vi "CreateWindow.vi"(8 "error in (no error)":errorcluster, 10 "Window Type":refnum<class "Window.lvclass">, 11 "Engine in":refnum<class "Engine.lvclass">) -> (0 "error out":errorcluster, 2 "Window Instance":refnum<class "Window.lvclass">, 3 "Engine out":refnum<class "Engine.lvclass">)   [LabVIEW 2020, in "GLF.lvlib" / "Engine.lvclass"]
uses:
  Engine.lvclass
  Engine.lvclass/Engine.ctl
  Window/Window.lvclass
  C:/Users/saukko/Dev/GLF/Sources/GLF/IUseDVRHandler/IUseDVRHandler.lvclass
  C:/Users/saukko/Dev/GLF/Sources/GLF/IAmGLF/IAmGLF.lvclass
  C:/Users/saukko/Dev/GLF/Sources/GLF/Window/Window.lvclass
  IAmGLF/IAmGLF.lvclass
  Command--enum.ctl
  Command-CreateWindow--cluster.ctl
  IAmGLF/InstanciationNotifierData--cluster.ctl
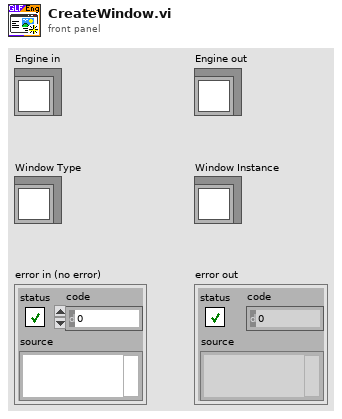
[diagram p1: front panel]
types:
  T1 = typedef "GLF.lvlib/IAmGLF.lvclass/InstanciationNotifierData--cluster.ctl" = cluster{"GLF Instance":refnum<class "IAmGLF.lvclass">, "Error":errorcluster}
  T2 = typedef "GLF.lvlib/Engine.lvclass/Command-CreateWindow--cluster.ctl" = cluster{"Window Type":refnum<class "Window.lvclass">, "Error Return Notifier":refnum<notifier>}
  T3 = typedef "GLF.lvlib/Engine.lvclass/Command--enum.ctl" = enum16{"Quit", "Create Window"}
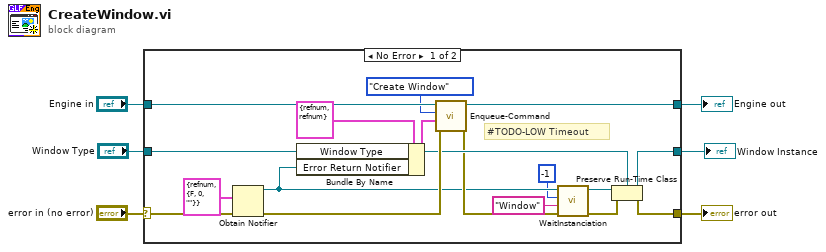
[diagram p0: block diagram]
diagram:
  n1 = case shown="No Error" "error in (no error)" {
    selector: "error in (no error)" -> [w19 w26]
    tunnel: [w9 w26] -> w5
    tunnel: [w22 w25] -> w3
    tunnel: "Engine in" -> [w23 w25]
    tunnel: "Window Type" -> [w15 w24]
    tunnel: [w16 w24] -> w1
    frame No Error {
      # "#TODO-LOW Timeout"
      n2 = Obtain Notifier(notification data type=T1 {"GLF Instance"=refnum, "Error"={"status"=FALSE, "code"=0, "source"=""}} ("Data"), error in (no error)=w19) -> (notifier out=w12:refnum<notifier>, error out=w20:errorcluster)  [unwired: 2 in, 1 out]
      n3 = Bundle By Name(cluster=T2 {"Window Type"=refnum, "Error Return Notifier"=refnum} ("Data"), "Window Type"=w15, "Error Return Notifier"=w12) -> (w17:T2)
      n4 = call "Enqueue-Command.vi"("error in (no error)"=w20, "Cmd Data"=w17, "Cmd"=Command--enum."Create Window", "Engine in"=w23) -> ("error out"=w13:errorcluster, "Engine out"=w22:refnum<class "Engine.lvclass">)  [unwired: 5 in, 1 out]
      n5 = call "WaitInstanciation.vi"("error in (no error)"=w13, "Timeout additional message (\"\")"="Window" ("Timeout additional message (\"\")"), "Timeout [ms]"=-1, "Instanciation Notifier"=w12) -> ("error out"=w10:errorcluster, "GLF Instance"=w11:refnum<class "IAmGLF.lvclass">)  [unwired: 6 in]
      n6 = Preserve Run-Time Class(object in=w11, error in=w10, 2:w15) -> (object out=w16:refnum<class "Window.lvclass">, error out=w9:errorcluster)
    }
    frame Error {
    }
  }
  "error out" <- w5
  "Engine out" <- w3
  "Window Instance" <- w1
